vi "Data Logging Pro.vi"() -> ()   [LabVIEW 2019]
uses:
  Controls/Data Button.ctl
  Controls/Chart Button.ctl
  <vilib>/DAQmx/read.llb/DAQmx Read (Analog 1D DBL NChan 1Samp).vi
  <vilib>/DAQmx/miscellaneous.llb/DAQmx Fill In Error Info.vi
  SubVIs/WSData.vi
  <vilib>/Platform/browser.llb/Open URL in Default Browser (string).vi
panel:
  out "ChartDataInput":enum16{"EUData", "RawData"}(ring)
  out "File Path":path
  out "ErrorLogging 2":errorcluster
  out "Current Time":string="2016-05-31 11:06:56"
  out "Data (EU)":dbl[](array[numeric]) format="%.2g"
  out "Data (Raw)":dbl[](array[numeric]) caption="Data (Raw Data, V)" format="%.2g"
  out "Database Connection":refnum<k7>
  out "ErrorLogging":errorcluster
  out "Exit":bool=TRUE
  out "Logging":bool
  out "Error Out":errorcluster
  in  "Error In":errorcluster
  out "DAQmx Task Name":refnum<k21>
  in  "Tab Control":enum32{"Chart", "Data"}(tab)
  in  "Open Data Window":T1
  in  "Open Chart Window":T2
  out "Waveform Chart":T3(graph)={"data[0]"=18.911298857159423, "data[1]"=59.99536966047508, "data[2]"=0.0, "data[3]"=0.0, "data[4]"=0.0, "data[5]"=0.0, "data[6]"=0.0, "data[7]"=0.0, "data[8]"=0.0}
  out "DataList":i32(listbox)=-1
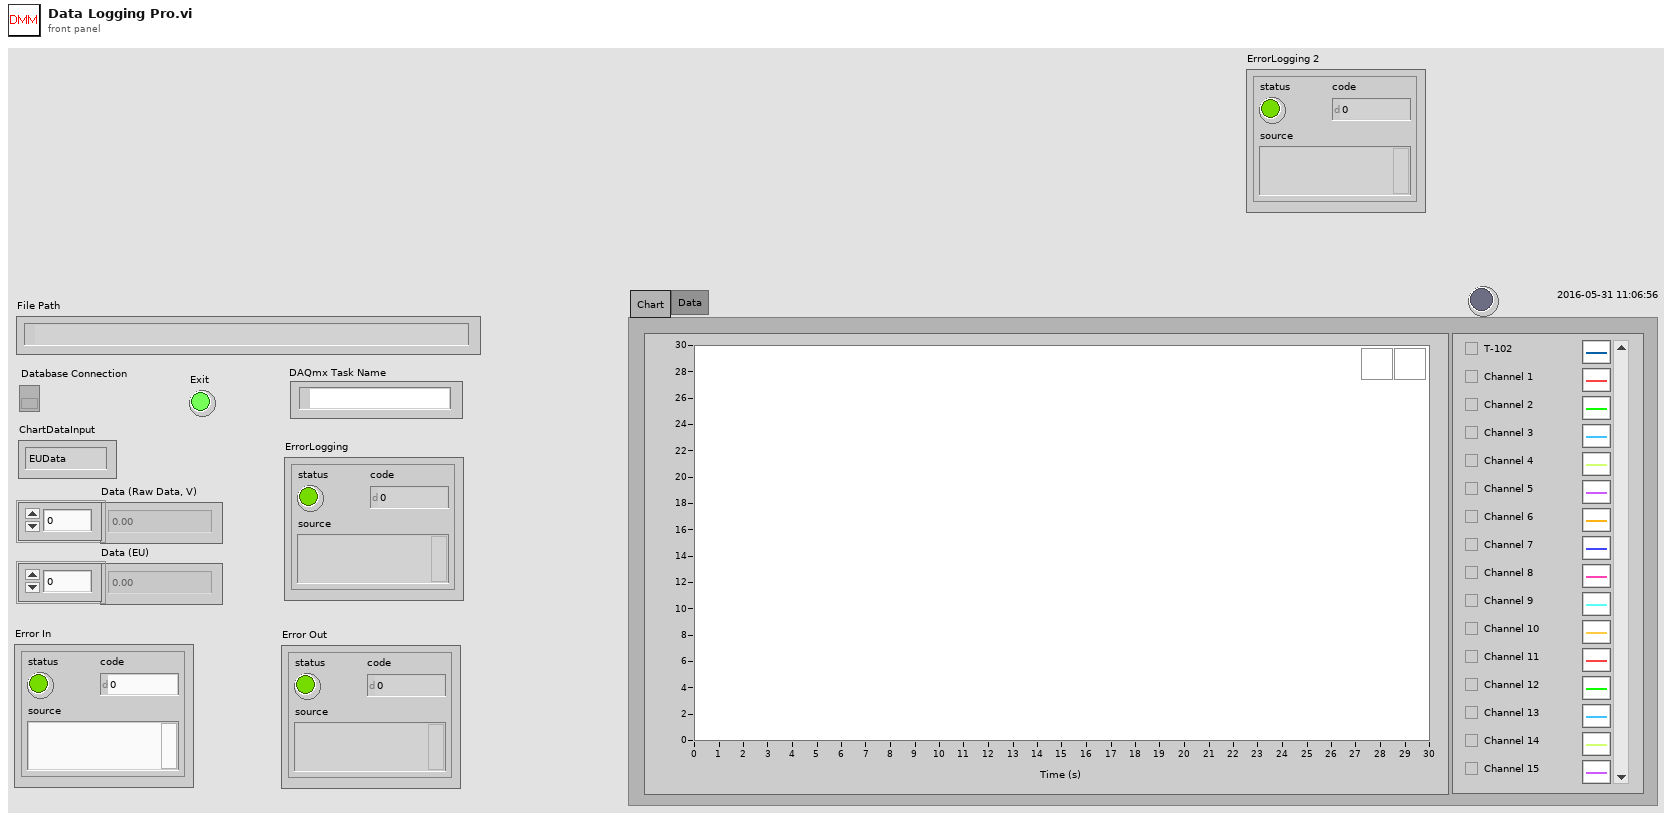
[diagram p1: front panel]
types:
  T1 = typedef "Data Button.ctl" = bool
  T2 = typedef "Chart Button.ctl" = bool
  T3 = cluster{"data[0]":dbl, "data[1]":dbl, "data[2]":dbl, "data[3]":dbl, "data[4]":dbl, "data[5]":dbl, "data[6]":dbl, "data[7]":dbl, "data[8]":dbl}
  T4 = typedef "Logging Settings.ctl" = cluster{"Logging Interval [s]":dbl, "Use Lowpass Filter":bool, "Tf [s]":dbl, "Logging Data to File":bool, "Log Folder":path, "Logging Data to Cloud Service":bool, "Data Cloud Service Url":string, "Use Random Data":bool}
  T5 = cluster{"TagId":string, "TagName":string, "TagType":string, "PhysicalChannel":tag, "Vmin":dbl, "Vmax":dbl, "Unit":string, "EUmin":dbl, "EUmax":dbl}[]
  T6 = cluster{"Data (Raw)[0]":dbl, "Data (Raw)[1]":dbl, "Data (Raw)[2]":dbl, "Data (Raw)[3]":dbl, "Data (Raw)[4]":dbl, "Data (Raw)[5]":dbl, "Data (Raw)[6]":dbl, "Data (Raw)[7]":dbl, "Data (Raw)[8]":dbl}
  T7 = cluster{"data[0]":dbl, "data[1]":dbl, "data[2]":dbl, "data[3]":dbl, "data[4]":dbl, "data[5]":dbl, "data[6]":dbl, "data[7]":dbl, "data[8]":dbl}[]
  T8 = enum32{"Bad", "Idle", "Run top level", "Running"}
  T9 = enum32{"Invalid", "Standard", "Closed", "Hidden", "Minimized", "Maximized"}
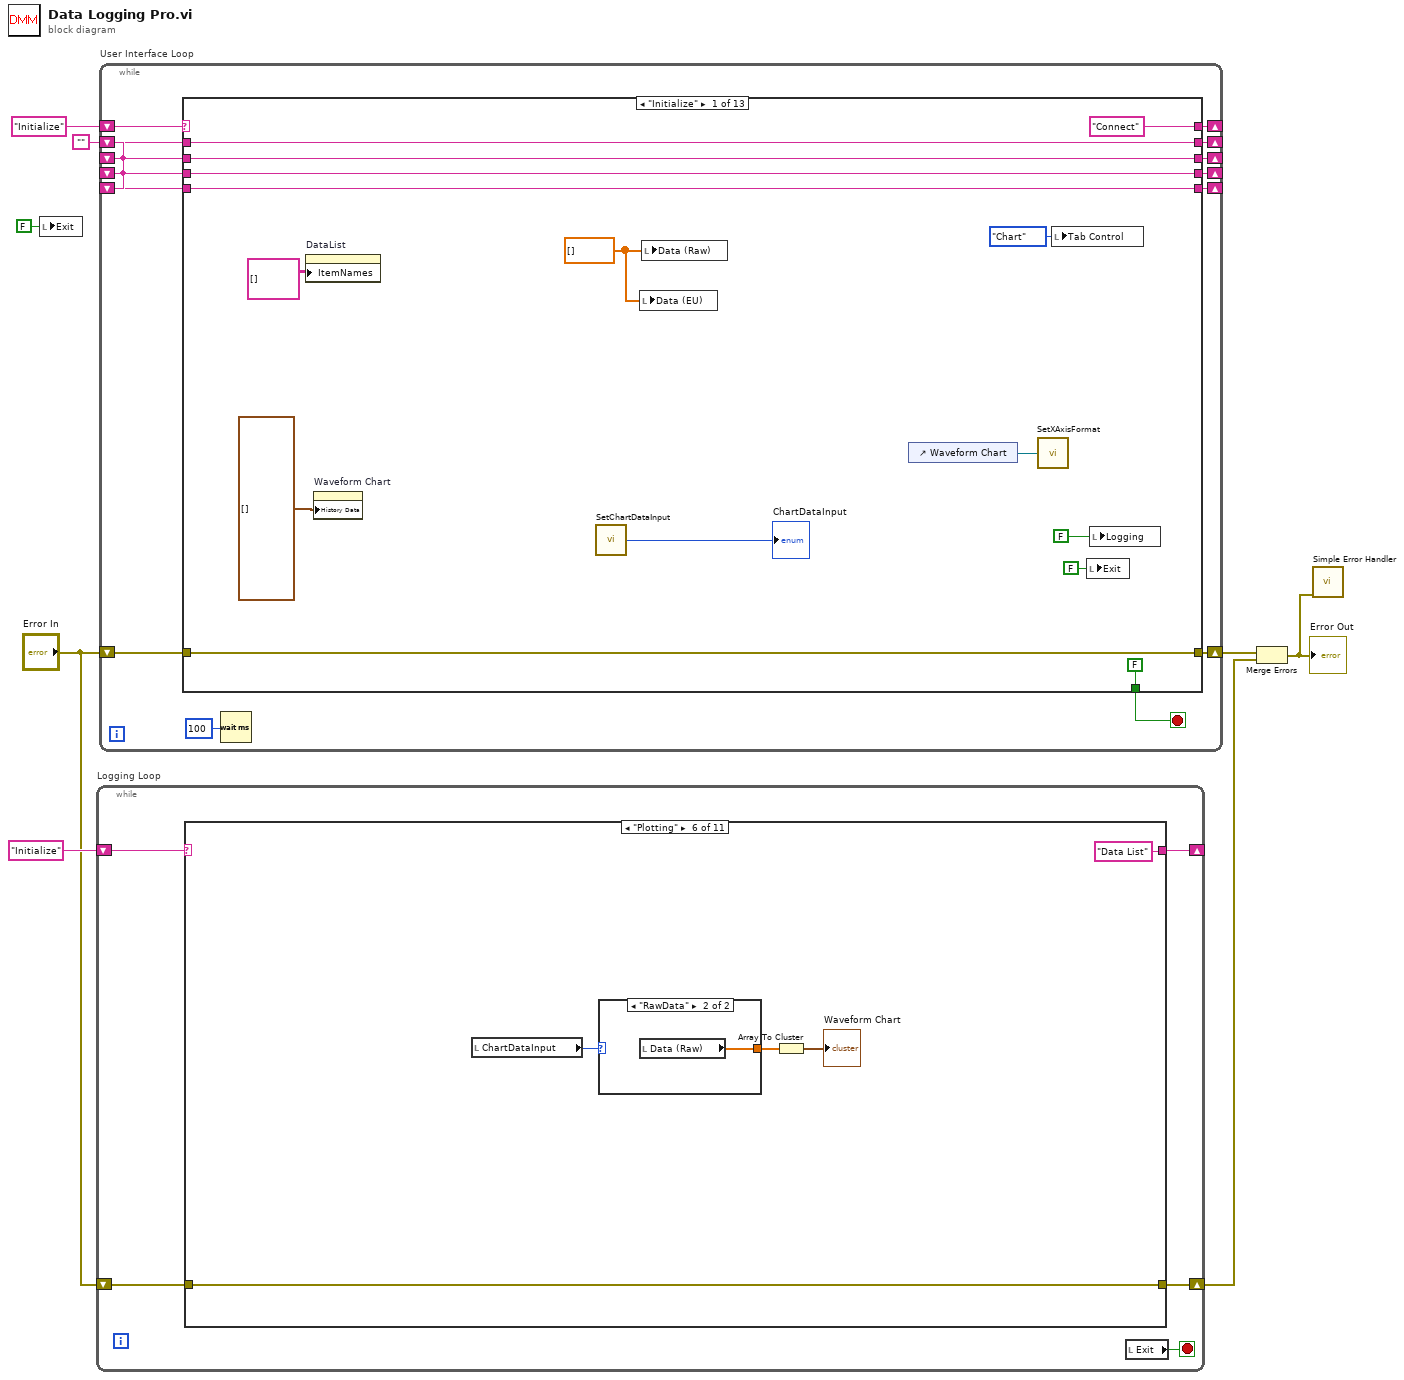
[diagram p0: block diagram]
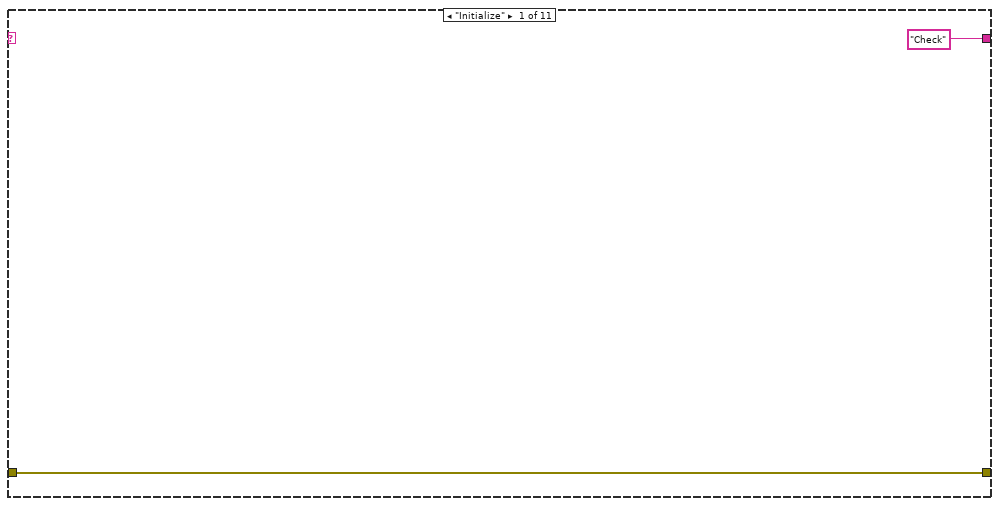
[diagram p2: hidden frame]
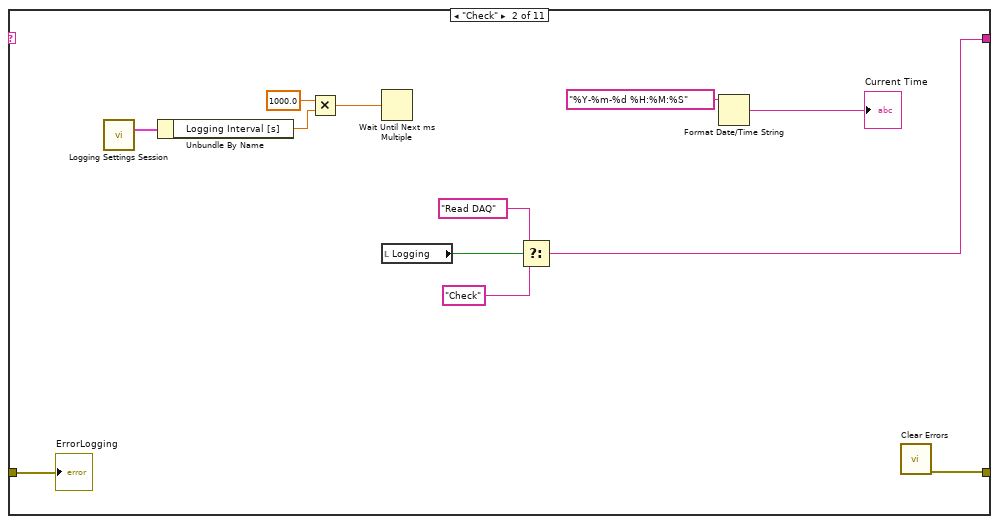
[diagram p3: hidden frame]
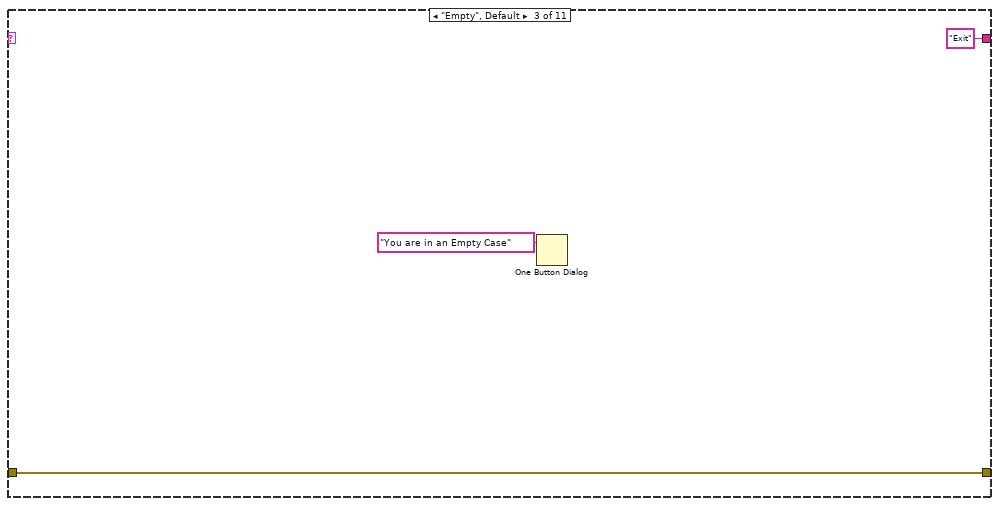
[diagram p4: hidden frame]
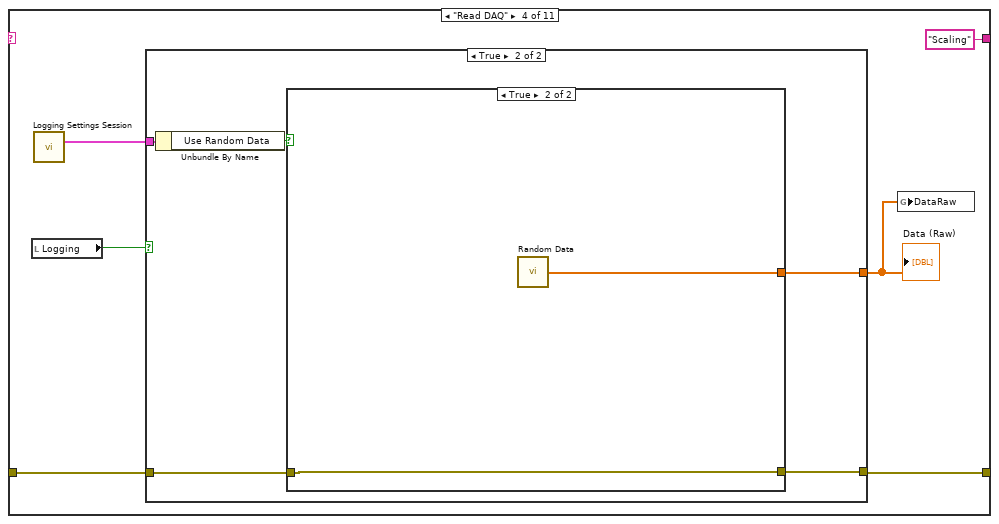
[diagram p5: hidden frame]
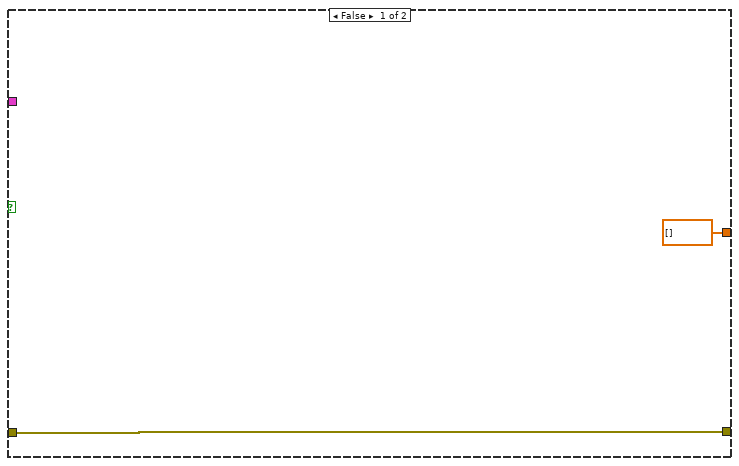
[diagram p6: hidden frame]
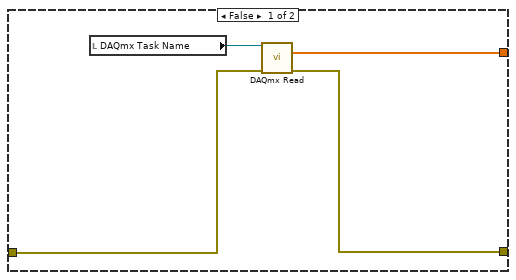
[diagram p7: hidden frame]
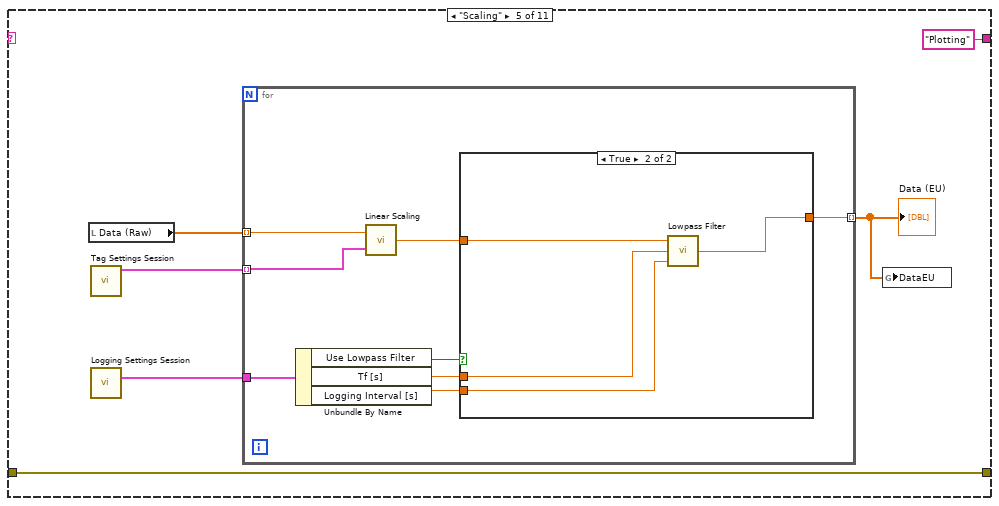
[diagram p8: hidden frame]
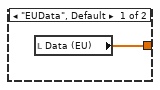
[diagram p10: hidden frame]
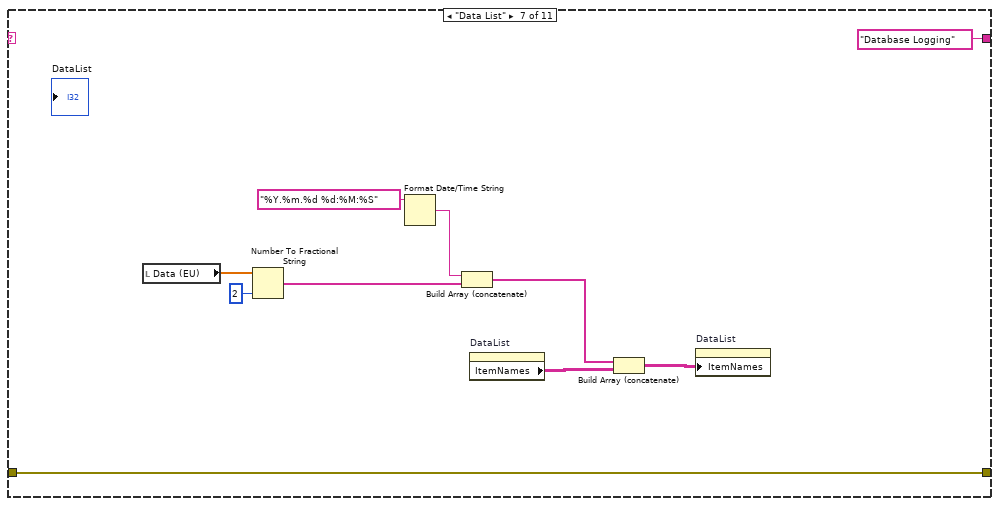
[diagram p11: hidden frame]
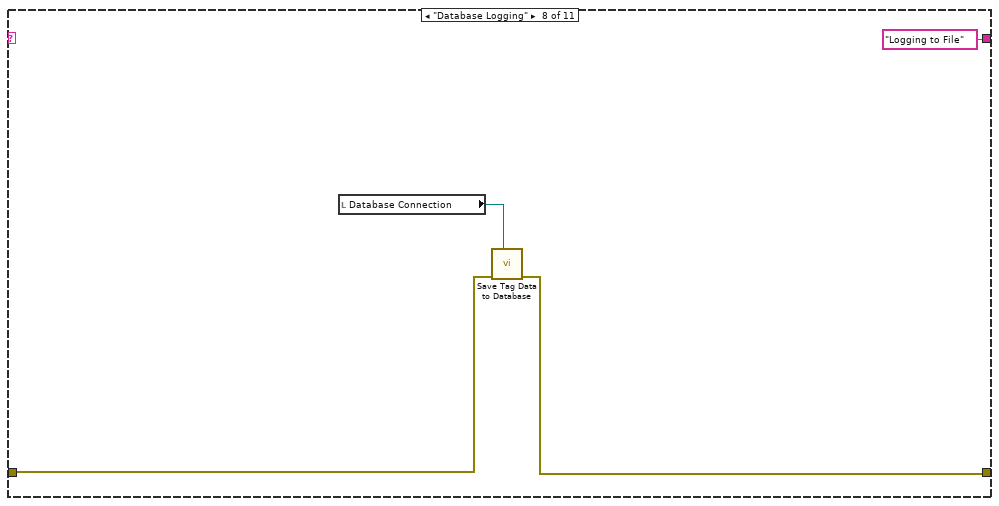
[diagram p12: hidden frame]
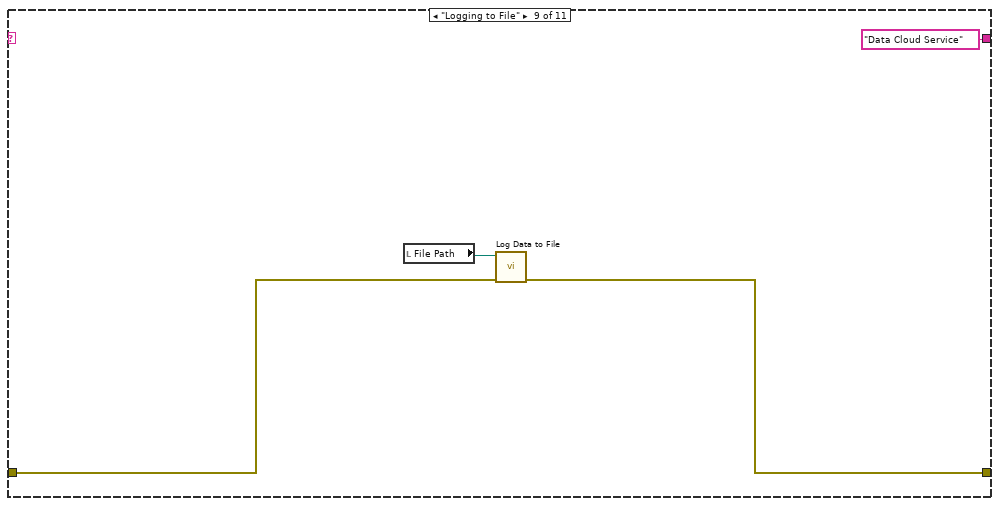
[diagram p13: hidden frame]
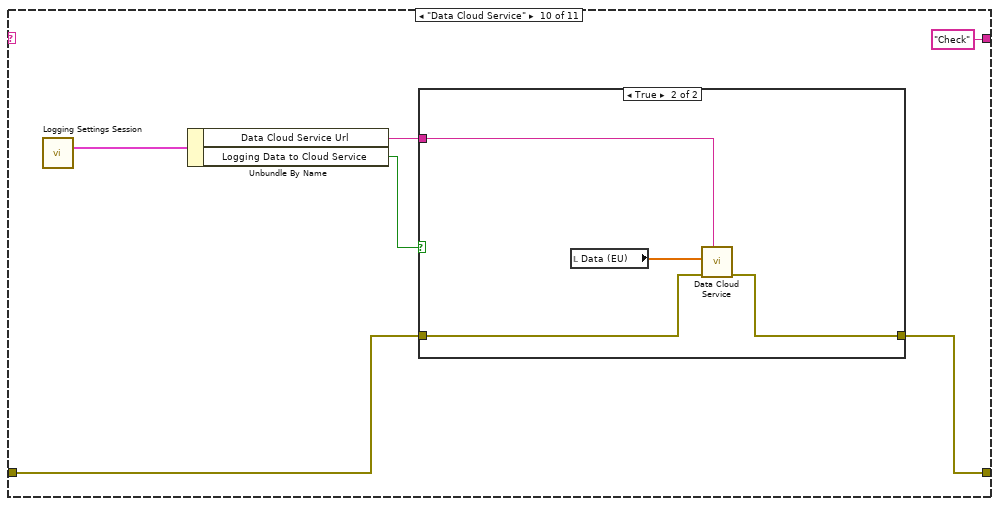
[diagram p14: hidden frame]
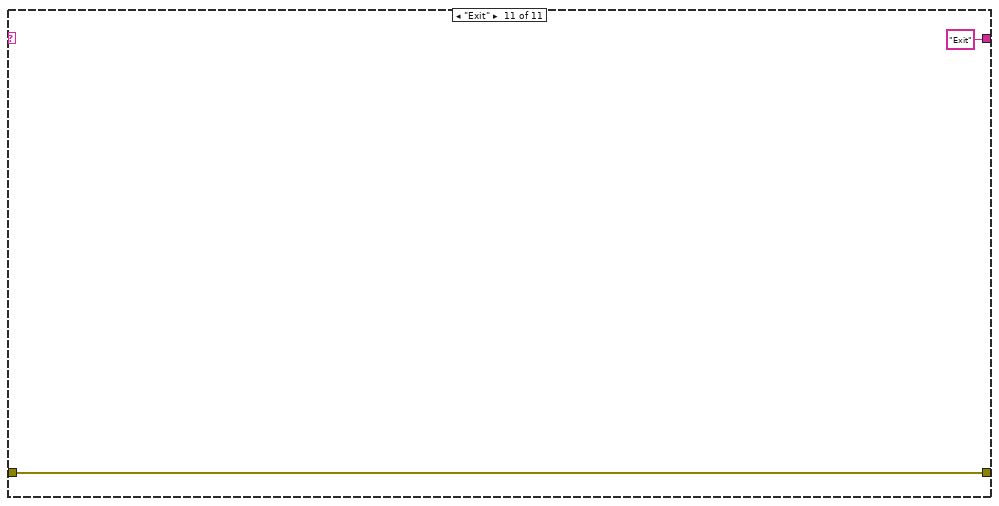
[diagram p16: hidden frame]
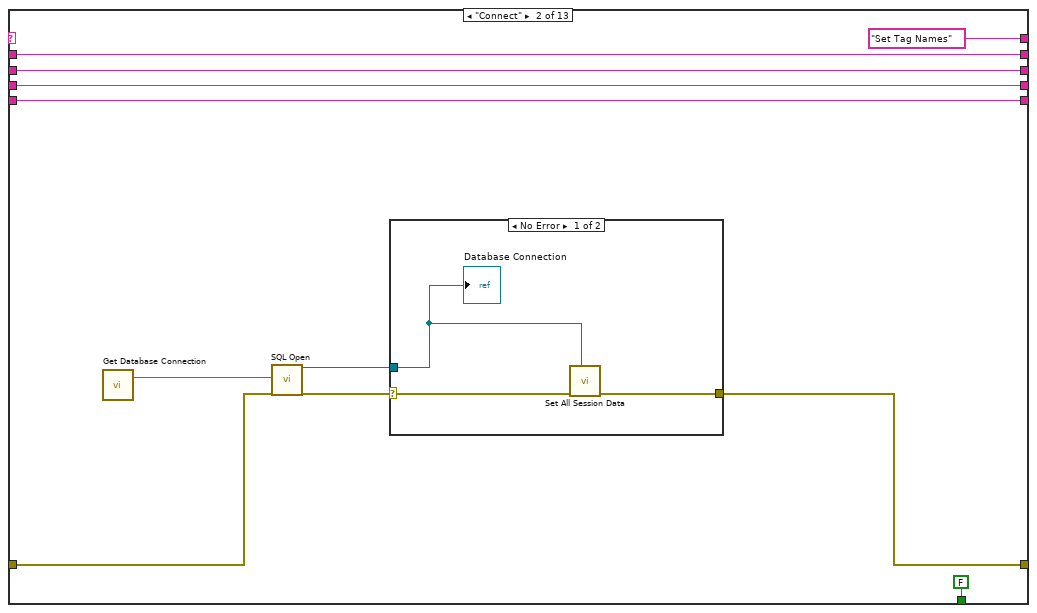
[diagram p17: hidden frame]
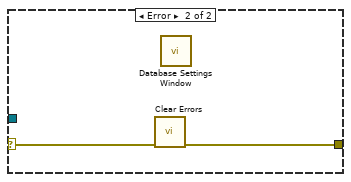
[diagram p18: hidden frame]
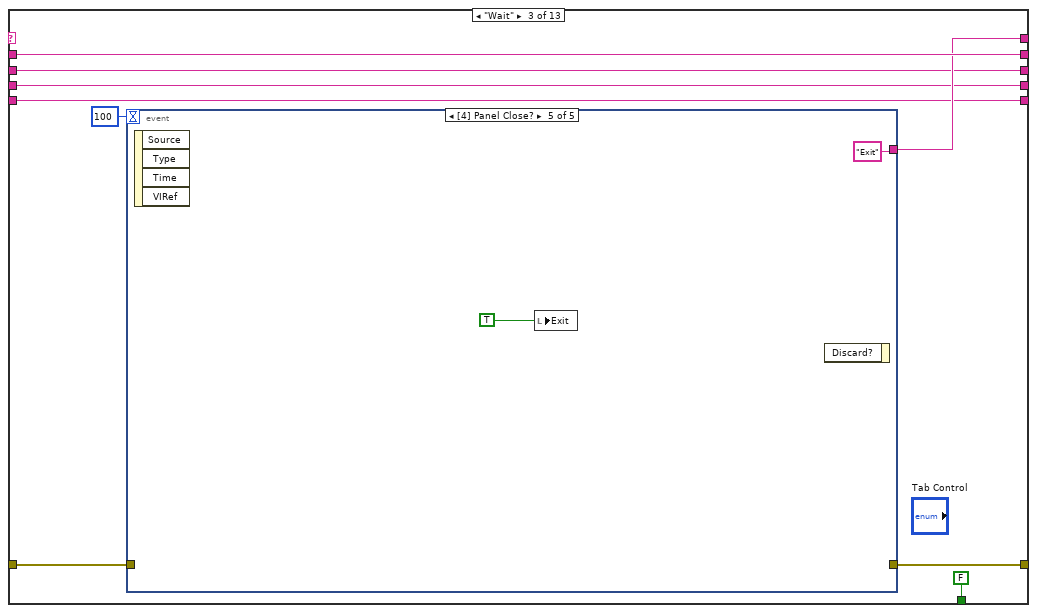
[diagram p19: hidden frame]
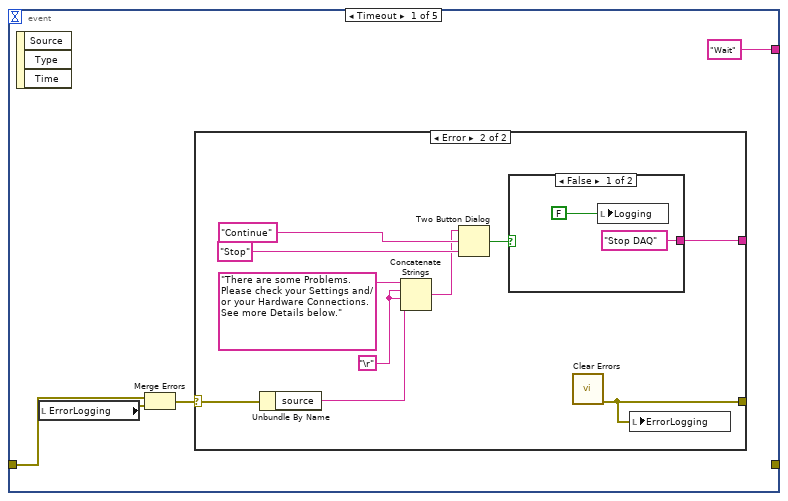
[diagram p20: hidden frame]
diagram:
  w7 = ""
  n1 = local write "Exit"(FALSE ("Exit")) -> ()
  n2 = while "Logging Loop" {
    shift-right: [w12] -> _
    shift-left: "Initialize" -> [w13]
    shift-right: [w9] -> w3
    shift-left: "Error In" -> [w10]
    stop <- w11 stop-if-true
    n3 = case shown="\"Plotting\"" w13 {
      tunnel: ["Check" w24 "Exit" "Scaling" "Plotting" "Data List" "Database Logging" "Logging to File" "Data Cloud Service" "Check" "Exit"] -> w12
      tunnel: w10 -> [w14 w22 w28 w35 w54 w72 w82 w88 w92 w98 w105]
      tunnel: [w14 w21 w28 w34 w54 w72 w82 w87 w91 w97 w105] -> w9
      frame "Initialize" {
      }
      frame "Check" {
        n4 = call "Logging Settings Session.vi"() -> ("Logging Settings"=w19:T4)  [unwired: 14 in, 1 out]
        n5 = Unbundle By Name(w19) -> ("Logging Interval [s]"=w18:dbl)
        n6 = Multiply(x=1000.0, y=w18) -> (x*y=w20:dbl)
        n7 = Wait Until Next ms Multiple(millisecond multiple=w20) -> ()  [unwired: 1 out]
        n8 = local read "Logging"() -> (w27:bool)
        n9 = Select(t="Read DAQ", s=w27, f="Check") -> (s? t:f=w24:string)
        n10 = Format Date/Time String(time format string (%c)="%Y-%m-%d %H:%M:%S") -> (date/time string=→"Current Time":string)  [unwired: 2 in]
        n11 = call <vilib>:"Clear Errors.vi"() -> ("error out"=w21:errorcluster)  [unwired: 6 in, 1 out]
        "ErrorLogging" <- w22
      }
      frame "Empty", Default {
        n12 = One Button Dialog(message="You are in an Empty Case") -> ()  [unwired: 1 in, 1 out]
      }
      frame "Read DAQ" {
        n13 = local read "Logging"() -> (w33:bool)
        n14 = call "Logging Settings Session.vi"() -> ("Logging Settings"=w31:T4)  [unwired: 14 in, 1 out]
        n15 = case shown="True" w33 {
          tunnel: w35 -> [w38 w42]
          tunnel: [w38 w41] -> w34
          tunnel: [dbl[] [] ("data") w43] -> w32
          tunnel: w31 -> [_ w40]
          frame False {
          }
          frame True {
            n16 = Unbundle By Name(w40) -> ("Use Random Data"=w39:bool)
            n17 = case shown="True" w39 {
              tunnel: [w46 w49] -> w43
              tunnel: w42 -> [w45 w48]
              tunnel: [w44 w48] -> w41
              frame False {
                n18 = local read "DAQmx Task Name"() -> (w47:refnum<k21>)
                n19 = call-poly <vilib>:"DAQmx Read.vi"("task/channels in"=w47, "error in"=w45) -> ("data"=w46:dbl[], "error out"=w44:errorcluster)  [unwired: 11 in, 1 out]
              }
              frame True {
                n20 = call "Random Data.vi"() -> ("Data"=w49:dbl[])  [unwired: 1 in]
              }
            }
          }
        }
        "Data (Raw)" <- w32
        n21 = global write "WSData.vi" "DataRaw"(w32) -> ()
      }
      frame "Scaling" {
        n22 = local read "Data (Raw)"() -> (w53:dbl[])
        n23 = call "Tag Settings Session.vi"() -> ("Tag Settings"=w51:T5)  [unwired: 10 in, 1 out]
        n24 = call "Logging Settings Session.vi"() -> ("Logging Settings"=w50:T4)  [unwired: 14 in, 1 out]
        n25 = for {
          tunnel: w53 -> [w63] mode=indexing
          tunnel: w51 -> [w62] mode=indexing
          tunnel: [w61] -> w52 mode=indexing
          tunnel: w50 -> [w56]
          n26 = Unbundle By Name(w56) -> ("Use Lowpass Filter"=w57:bool, "Tf [s]"=w59:dbl, "Logging Interval [s]"=w58:dbl)
          n27 = call "Linear Scaling.vi"("Tag"=w62, "x"=w63) -> ("y"=w60:dbl)
          n28 = case shown="True" w57 {
            tunnel: w60 -> [w64 w68]
            tunnel: [w64 w67] -> w61
            tunnel: w59 -> [_ w66]
            tunnel: w58 -> [_ w65]
            frame False {
            }
            frame True {
              n29 = call "Lowpass Filter.vi"("Ts [s]"=w65, "Tf [s]"=w66, "Filter Input"=w68) -> ("Filter Output"=w67:dbl)
            }
          }
        }
        "Data (EU)" <- w52
        n30 = global write "WSData.vi" "DataEU"(w52) -> ()
      }
      frame "Plotting" {
        n31 = local read "ChartDataInput"() -> (w70:enum16{"EUData", "RawData"})
        n32 = case shown="\"RawData\"" w70 {
          tunnel: [w74 w75] -> w69
          frame "EUData", Default {
            n33 = local read "Data (EU)"() -> (w74:dbl[])
          }
          frame "RawData" {
            n34 = local read "Data (Raw)"() -> (w75:dbl[])
          }
        }
        n35 = Array To Cluster(array=w69) -> (cluster=→"Waveform Chart":T6)
      }
      frame "Data List" {
        n36 = local read "Data (EU)"() -> (w84:dbl[])
        n37 = Number To Fractional String(number=w84, precision (6)=i16 2) -> (F-format string=w79:string[])  [unwired: 2 in]
        n38 = Format Date/Time String(time format string (%c)="%Y.%m.%d %d:%M:%S") -> (date/time string=w80:string)  [unwired: 2 in]
        n39 = Build Array (concatenate) "Build Array"(w80, w79) -> (w76:string[])
        n40 = property on="DataList" class="MCListbox (strict)"() -> ("ItemNames"=w77:string[][])  [unwired: 2 in, 2 out]
        n41 = Build Array (concatenate) "Build Array"(w76, w77) -> (w83:string[][])
        n42 = property on="DataList" class="MCListbox (strict)"("ItemNames"=w83) -> ()  [unwired: 2 in, 2 out]
      }
      frame "Database Logging" {
        n43 = local read "Database Connection"() -> (w86:refnum<k7>)
        n44 = call "Save Tag Data to Database.vi"("Database Connection"=w86, "Error In"=w88) -> ("Error Out"=w87:errorcluster)  [unwired: 9 in]
      }
      frame "Logging to File" {
        n45 = local read "File Path"() -> (w90:path)
        n46 = call "Log Data to File.vi"("Error In"=w92, "Log File Path"=w90) -> ("Error Out"=w91:errorcluster)  [unwired: 9 in]
      }
      frame "Data Cloud Service" {
        n47 = call "Logging Settings Session.vi"() -> ("Logging Settings"=w94:T4)  [unwired: 14 in, 1 out]
        n48 = Unbundle By Name(w94) -> ("Data Cloud Service Url"=w96:string, "Logging Data to Cloud Service"=w95:bool)
        n49 = case shown="True" w95 {
          tunnel: w98 -> [w100 w104]
          tunnel: [w100 w103] -> w97
          tunnel: w96 -> [_ w101]
          frame False {
          }
          frame True {
            n50 = local read "Data (EU)"() -> (w102:dbl[])
            n51 = call "Data Cloud Service.vi"("Data Cloud Service Url"=w101, "Error In"=w104, "Data (EU)"=w102) -> ("Error Out"=w103:errorcluster)  [unwired: 8 in]
          }
        }
      }
      frame "Exit" {
      }
    }
    n52 = local read "Exit"() -> (w11:bool)
  }
  n53 = while "User Interface Loop" {
    shift-right: [w118] -> _
    shift-left: "Initialize" -> [w120]
    shift-right: [w116] -> _
    shift-left: w7 -> [w117]
    shift-right: [w113] -> _
    shift-left: w7 -> [w114]
    shift-right: [w111] -> _
    shift-left: w7 -> [w112]
    shift-right: [w109] -> _
    shift-left: w7 -> [w110]
    shift-right: [w107] -> w2
    shift-left: "Error In" -> [w108]
    stop <- w115 stop-if-true
    n54 = case shown="\"Initialize\"" w120 {
      tunnel: ["Connect" "Set Tag Names" w158 "Exit" "Connect" "Wait" "Wait" "Set Tag Names" "Wait" "Wait" "Wait" "Wait" "Exit"] -> w118
      tunnel: w117 -> [w134 w146 w159 w265 w272 w283 w308 w317 w328 w343 w353 w362 w372]
      tunnel: [w134 w146 w159 w265 w272 w283 w308 w317 w328 w343 w353 w362 w372] -> w116
      tunnel: [FALSE FALSE FALSE FALSE FALSE FALSE FALSE FALSE FALSE FALSE FALSE FALSE TRUE] -> w115
      tunnel: w114 -> [w132 w144 w156 w262 w270 w281 w306 w315 w326 w341 w351 w360 w370]
      tunnel: [w132 w144 w156 w262 w270 w281 w306 w315 w326 w341 w351 w360 w370] -> w113
      tunnel: w112 -> [w131 w143 w155 w261 w269 w280 w305 w314 w325 w340 w350 w359 w369]
      tunnel: [w131 w143 w155 w261 w269 w280 w305 w314 w325 w340 w350 w359 w369] -> w111
      tunnel: w110 -> [w130 w142 w154 w260 w268 w279 w304 w313 w324 w339 w349 w358 w368]
      tunnel: [w130 w142 w154 w260 w268 w279 w304 w313 w324 w339 w349 w358 w368] -> w109
      tunnel: w108 -> [w123 w139 w153 w259 w267 w277 w302 w310 w319 w337 w347 w355 w367]
      tunnel: [w123 w136 w152 w259 w267 w277 w301 w309 w318 w336 w346 w354 w367] -> w107
      frame "Initialize" {
        w126 = dbl[] [] ("Data")
        n55 = property on="DataList" class="MCListbox (strict)"("ItemNames"=string[][] [] ("Item Names")) -> ()  [unwired: 2 in, 2 out]
        n56 = property on="Waveform Chart" class="WFChart (strict)"("History Data"=T7 []) -> ()  [unwired: 2 in, 2 out]
        n57 = call "SetChartDataInput.vi"() -> ("ChartDataInput"=→"ChartDataInput":enum16{"EUData", "RawData"})  [unwired: 1 in]
        n58 = local write "Data (EU)"(w126) -> ()
        n59 = local write "Data (Raw)"(w126) -> ()
        n60 = control-ref of="Waveform Chart"() -> (w122:refnum<vi>)
        n61 = call "SetXAxisFormat.vi"("Waveform Chart Reference"=w122) -> ()  [unwired: 1 in]
        n62 = local write "Tab Control"(enum32{"Chart", "Data", "Logging", "Help"}."Chart" ("Tab Control")) -> ()
        n63 = local write "Exit"(FALSE ("Exit")) -> ()
        n64 = local write "Logging"(FALSE ("Logging")) -> ()
      }
      frame "Connect" {
        n65 = call "Get Database Connection.vi"() -> ("Database  Connection String"=w138:string)  [unwired: 2 in, 1 out]
        n66 = call <vilib>:"SQL Open.vi"("ConnectionString In"=w138, "Error in (no error)"=w139) -> ("Connection Out"=w140:refnum<k7>, "Error out"=w137:errorcluster)  [unwired: 16 in]
        n67 = case shown="No Error" w137 {
          selector: w137 -> [w149 w151]
          tunnel: w140 -> [w147 _]
          tunnel: [w148 w150] -> w136
          frame No Error {
            n68 = call "Set All Session Data.vi"("Database Connection"=w147, "Error In"=w149) -> ("Error Out"=w148:errorcluster)  [unwired: 9 in]
            "Database Connection" <- w147
          }
          frame Error {
            n69 = call <vilib>:"Clear Errors.vi"("error in (no error)"=w151) -> ("error out"=w150:errorcluster)  [unwired: 5 in, 1 out]
            n70 = call "Database Settings Window.vi"() -> ()  [unwired: 12 in]
          }
        }
      }
      frame "Wait" {
        n71 = event shown="[4] Panel Close?" {
          selector: _ -> [_ _ _ _ _]
          dyn-events: _ -> [_ _ _ _ _]
          timeout: 100 -> [_ _ _ _ _]
          tunnel: ["Wait" "Wait" "Wait" w202 "Exit"] -> w158
          tunnel: w153 -> [w162 _ _ w200 _]
          tunnel: [_ _ _ w199 _] -> w152
          event Timeout {
            n72 = event-data() -> ()  [unwired: 1 in, 3 out]
            n73 = local read "ErrorLogging"() -> (w163:errorcluster)
            n74 = Merge Errors(w162, w163) -> (w161:errorcluster)
            n75 = case shown="Error" w161 {
              selector: w161 -> [w166 w172]
              tunnel: [w166 w167] -> _
              tunnel: ["Wait" w176] -> _
              frame No Error {
              }
              frame Error {
                w169 = "\r"
                n76 = Unbundle By Name(w172) -> ("source"=w168:string)
                n77 = Concatenate Strings("There are some Problems. Please check your Settings and/or your Hardware Connections. See more Details below." ("message"), w169, w169, w168) -> (w170:string)
                n78 = Two Button Dialog(message=w170, 1:"Stop" ("F button name (\"Cancel\")"), 2:"Continue" ("T button name (\"OK\")")) -> (T button?=w173:bool)
                n79 = case shown="False" w173 {
                  tunnel: ["Stop DAQ" "Wait"] -> w176
                  frame False {
                    n80 = local write "Logging"(FALSE ("Logging")) -> ()
                  }
                  frame True {
                  }
                }
                n81 = call <vilib>:"Clear Errors.vi"() -> ("error out"=w167:errorcluster)  [unwired: 6 in, 1 out]
                n82 = local write "ErrorLogging"(w167) -> ()
              }
            }
          }
          event Value Change {
            n83 = event-data() -> ()  [unwired: 1 in, 6 out]
            n84 = vi-ref "Data Window.vi"() -> (w180:refnum<vi>)
            n85 = property class="VI"(reference=w180) -> ("Exec.State"=w183:T8)  [unwired: 1 in, 2 out]
            n86 = Equal?(x=w183, y=T8."Idle" ("Execution:State")) -> (x = y?=w181:bool)
            n87 = case shown="True" w181 {
              tunnel: w180 -> [_ w185]
              frame False {
              }
              frame True {
                n88 = invoke class="VI" method="Run VI"(reference=w185, "Wait until done"=FALSE ("Wait Until Done"), "Auto Dispose Ref"=TRUE ("Auto Dispose Reference")) -> (reference out=w186:refnum<vi>)  [unwired: 2 in, 4 out]
                n89 = invoke class="VI" method="FP.Open"(reference=w186) -> ()  [unwired: 4 in, 5 out]
              }
            }
          }
          event Value Change {
            n90 = event-data() -> ()  [unwired: 1 in, 6 out]
            n91 = vi-ref "Chart Window.vi"() -> (w189:refnum<vi>)
            n92 = property class="VI"(reference=w189) -> ("Exec.State"=w191:T8)  [unwired: 1 in, 2 out]
            n93 = Equal?(x=w191, y=T8."Idle" ("Execution:State")) -> (x = y?=w193:bool)
            n94 = case shown="True" w193 {
              tunnel: w189 -> [_ w195]
              frame False {
              }
              frame True {
                n95 = invoke class="VI" method="Run VI"(reference=w195, "Wait until done"=FALSE ("Wait Until Done"), "Auto Dispose Ref"=TRUE ("Auto Dispose Reference")) -> (reference out=w196:refnum<vi>)  [unwired: 2 in, 4 out]
                n96 = invoke class="VI" method="FP.Open"(reference=w196, "State"=T9."Maximized") -> ()  [unwired: 3 in, 5 out]
              }
            }
          }
          event Menu Selection (User) {
            n97 = event-data() -> ("MenuRef"=w201:refnum<k9>, "ItemTag"=w203:string)  [unwired: 1 in, 5 out]
            n98 = case shown="\"Exit\"" w203 {
              tunnel: ["Wait" "Exit" "Database Settings" "Device Settings" "Tag Settings" "Logging Settings" "Initialize DAQ" "Stop DAQ" "Wait" "Wait" "Wait" "Wait"] -> w202
              tunnel: w201 -> [_ _ _ _ _ _ w226 w229 _ _ _ _]
              tunnel: w200 -> [w204 w207 w209 w211 w213 w215 w223 w231 w242 w247 w250 w253]
              tunnel: [w204 w207 w209 w211 w213 w215 w217 w230 w242 w247 w250 w253] -> w199
              frame "None", Default {
              }
              frame "Exit" {
                "Exit" <- TRUE ("Exit")
              }
              frame "Database Settings" {
              }
              frame "Device Settings" {
              }
              frame "Tag Settings" {
              }
              frame "Logging Settings" {
              }
              frame "Start DAQ" {
                n99 = Set Menu Item Info(6:TRUE ("checked"), 7:"Start DAQ" ("item tag"), 8:w223, 9:FALSE ("enabled"), 11:w226) -> (0:w218:errorcluster, 3:w219:refnum<k9>)  [unwired: 2 in]
                n100 = Set Menu Item Info(6:FALSE ("checked"), 7:"Stop DAQ" ("item tag"), 8:w218, 9:TRUE ("enabled"), 11:w219) -> (0:w217:errorcluster)  [unwired: 2 in, 1 out]
              }
              frame "Stop DAQ" {
                n101 = local write "Logging"(FALSE ("Logging")) -> ()
                n102 = Set Menu Item Info(6:FALSE ("checked"), 7:"Start DAQ" ("item tag"), 8:w231, 9:TRUE ("enabled"), 11:w229) -> (0:w232:errorcluster, 3:w233:refnum<k9>)  [unwired: 2 in]
                n103 = Set Menu Item Info(6:FALSE ("checked"), 7:"Stop DAQ" ("item tag"), 8:w232, 9:FALSE ("enabled"), 11:w233) -> (0:w230:errorcluster)  [unwired: 2 in, 1 out]
              }
              frame "User Guide" {
                n104 = call <vilib>:"Application Directory.vi"() -> ("Application Directory"=w245:path)
                n105 = Build Path(base path=w245, name or relative path="Datalogging and Monitoring Pro User Guide.pdf" ("URL")) -> (appended path=w243:path)
                n106 = call <vilib>:"Open Acrobat Document.vi"("acrobat document"=w243) -> ()  [unwired: 6 in, 1 out]
              }
              frame "Video" {
                n107 = call-poly <vilib>:"Open URL in Default Browser.vi"("URL"="https://www.youtube.com/playlist?list=PLdb-TcK6Aqj3qcbxD6N5TChz8UNxxyRSs") -> ()  [unwired: 5 in, 2 out]
              }
              frame "Data Dashboard for LabVIEW" {
                n108 = call-poly <vilib>:"Open URL in Default Browser.vi"("URL"="https://www.ni.com/mobile/") -> ()  [unwired: 5 in, 2 out]
              }
              frame "Home" {
                n109 = call-poly <vilib>:"Open URL in Default Browser.vi"("URL"="http://home.hit.no/~hansha/") -> ()  [unwired: 5 in, 2 out]
              }
            }
          }
          event Panel Close? {
            n110 = event-data() -> ()  [unwired: 1 in, 4 out]
            n111 = local write "Exit"(TRUE ("Exit")) -> ()
            n112 = event-data() -> ()  [unwired: 2 in, 1 out]
          }
        }
      }
      frame "Empty", Default {
        n113 = One Button Dialog(message="You are in an Empty Case") -> ()  [unwired: 1 in, 1 out]
      }
      frame "Database Settings" {
        n114 = call "Database Settings Window.vi"() -> ()  [unwired: 12 in]
      }
      frame "Set Tag Names" {
        n115 = call "Tag Settings Session.vi"() -> ("Tag Settings"=w274:T5)  [unwired: 10 in, 1 out]
        n116 = for {
          tunnel: w274 -> [w290] mode=indexing
          tunnel: [w284] -> w273 mode=indexing
          i -> [w291]
          n117 = Unbundle By Name(w290) -> ("TagName"=w289:string, "Unit"=w285:string)
          n118 = Empty String/Path?(string/path=w289) -> (empty?=w293:bool)
          n119 = property on="Waveform Chart" class="WFChart (strict)"("Active Plot"=w291) -> (error out=w295:errorcluster)  [unwired: 2 in, 1 out]
          n120 = case shown="True" w293 {
            tunnel: [w296 w297] -> w292
            tunnel: w289 -> [w296 _]
            tunnel: w291 -> [_ w299]
            frame False {
            }
            frame True {
              n121 = Number To Decimal String(number=w299) -> (decimal integer string=w298:string)  [unwired: 1 in]
              n122 = Concatenate Strings("Channel " ("string"), w298) -> (w297:string)
            }
          }
          n123 = String Subset(string=w292, length (rest)=11 ("length (rest)")) -> (substring=w286:string)  [unwired: 1 in]
          n124 = property on="Waveform Chart" class="WFChart (strict)"(error in=w295, "Plot.Plot Name"=w286) -> ()  [unwired: 1 in, 2 out]
          n125 = Concatenate Strings(w286, " [" ("string"), w285, "]" ("string")) -> (w284:string)
        }
        n126 = Build Array (concatenate)("Date & Time", w273) -> (w275:string[])
        n127 = property on="DataList" class="MCListbox (strict)"("ColHdrString"=w275) -> ()  [unwired: 2 in, 2 out]
      }
      frame "Device Settings" {
        n128 = call "Device Settings Window.vi"("Error In"=w302) -> ("Error Out"=w301:errorcluster)  [unwired: 10 in]
      }
      frame "Tag Settings" {
        n129 = local read "Database Connection"() -> (w311:refnum<k7>)
        n130 = call "Tag Settings Window.vi"("Error In"=w310, "Database Connection"=w311) -> ("Error Out"=w309:errorcluster)  [unwired: 9 in]
      }
      frame "Logging Settings" {
        n131 = call "Logging Settings Window.vi"("Error In"=w319) -> ("Error Out"=w320:errorcluster)  [unwired: 10 in]
        n132 = call "Logging Settings Session.vi"("Error In"=w320) -> ("Logging Settings"=w321:T4, "Error Out"=w318:errorcluster)  [unwired: 13 in]
        n133 = Unbundle By Name(w321) -> ("Logging Interval [s]"=w322:dbl)
        n134 = property on="Waveform Chart" class="WFChart (strict)"("XScale.Multiplier"=w322) -> ()  [unwired: 2 in, 2 out]
      }
      frame "Initialize DAQ" {
        n135 = call "DAQ Initialize.vi"("error in"=w337) -> ("error out"=w336:errorcluster, "DAQmx Task Name"=→"DAQmx Task Name":refnum<k21>)  [unwired: 9 in]
        n136 = case shown="No Error" w336 {
          frame No Error {
            "Logging" <- TRUE ("Logging")
          }
          frame Error {
          }
        }
        n137 = call "Logging Settings Session.vi"() -> ("Logging Settings"=w331:T4)  [unwired: 14 in, 1 out]
        n138 = Unbundle By Name(w331) -> ("Log Folder"=w330:path, "Logging Interval [s]"=w333:dbl)
        n139 = property on="DataList" class="MCListbox (strict)"("ItemNames"=string[][] [] ("Item Names")) -> ()  [unwired: 2 in, 2 out]
        n140 = property on="Waveform Chart" class="WFChart (strict)"("XScale.Multiplier"=w333) -> ()  [unwired: 2 in, 2 out]
        n141 = call "Create File Path.vi"("Folder Path"=w330) -> ("File Path"=→"File Path":path)
        n142 = property on="Waveform Chart" class="WFChart (strict)"("History Data"=T7 []) -> ()  [unwired: 2 in, 2 out]
      }
      frame "Stop DAQ" {
        n143 = local read "DAQmx Task Name"() -> (w348:refnum<k21>)
        n144 = call <vilib>:"DAQmx Clear Task.vi"("task in"=w348, "error in"=w347) -> ("error out"=w346:errorcluster)  [unwired: 13 in]
      }
      frame "Disconnect from Database" {
        n145 = local read "Database Connection"() -> (w356:refnum<k7>)
        n146 = call <vilib>:"SQL Close.vi"("Connection In"=w356, "Error in (no error)"=w355) -> ("Error out"=w354:errorcluster)  [unwired: 17 in]
      }
      frame "Exit" {
        w364 = dbl[] [] ("Data")
        n147 = local write "Data (EU)"(w364) -> ()
        n148 = local write "Data (Raw)"(w364) -> ()
        n149 = local write "Logging"(FALSE ("Logging")) -> ()
        n150 = call "Check if Executable program.vi"() -> ("Exe?"=w363:bool)  [unwired: 1 in]
        n151 = case shown="True" w363 {
          frame False {
            n152 = Stop(stop? (T)=TRUE) -> ()
          }
          frame True {
            n153 = Quit LabVIEW(quit? (T)=TRUE) -> ()
          }
        }
      }
    }
    n154 = Wait (ms)(milliseconds to wait=u32 100 ("millisecond timer value")) -> ()  [unwired: 1 out]
  }
  n155 = Merge Errors(w2, w3) -> (w1:errorcluster)
  "Error Out" <- w1
  n156 = call <vilib>:"Simple Error Handler.vi"("error in (no error)"=w1) -> ()  [unwired: 4 in, 5 out]
